vi "Fix up file date time to whats in file name.vi"(8 "error in":errorcluster) -> (0 "error out":errorcluster, 2 "Selected folder path":string, 3 "File path names":string[](array[string]))   [LabVIEW 2013]
panel:
  in  "Fix create date? (y)":bool=TRUE
  out "standard error":string
  out "standard output":string
  out "cmd shell cmds":string[](array[string])
  out "Records":i32
  # "Modified is false"
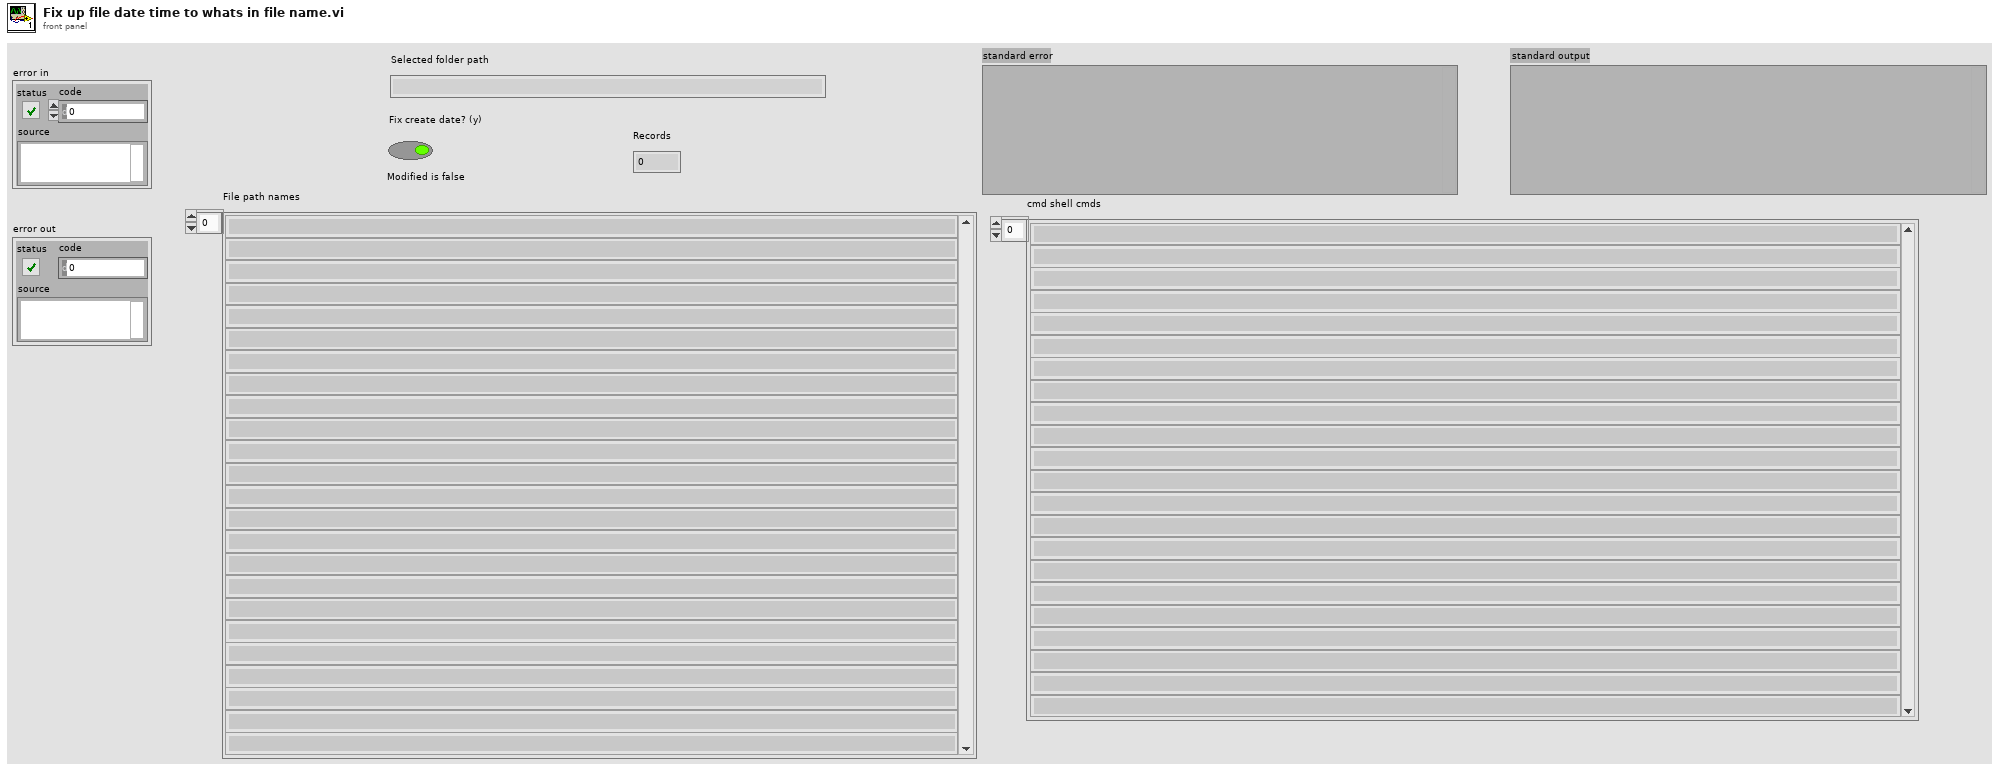
[diagram p1: front panel]
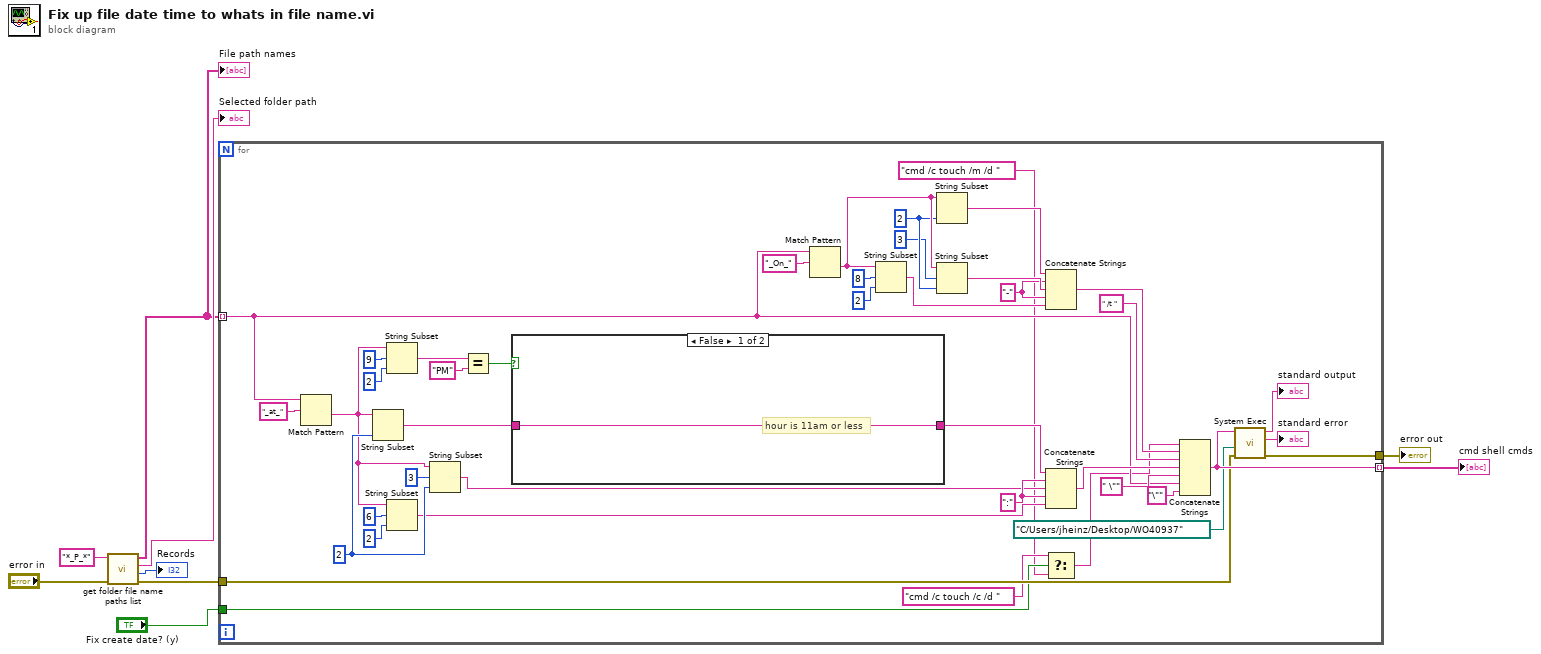
[diagram p0: block diagram]
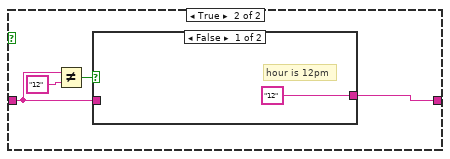
[diagram p2: hidden frame]
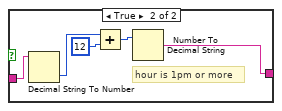
[diagram p3: hidden frame]
diagram:
  n1 = call "get folder file name paths list.vi"("error in"="error in", "file search pattern"="*_P_*") -> ("error out"=w4:errorcluster, "Records"=→"Records":i32, "Selected folder path"=→"Selected folder path":string, "File path names"=w5:string[])  [unwired: 6 in]
  "File path names" <- w5
  n2 = for {
    tunnel: w5 -> [w21] mode=indexing
    tunnel: w4 -> [w18]
    tunnel: [w17] -> w3
    tunnel: [w19] -> w2 mode=indexing
    tunnel: "Fix create date? (y)" -> [w13]
    w34 = ":" ("string")
    w37 = 2 ("length (rest)")
    w43 = "-" ("string")
    w49 = 2 ("length (rest)")
    n3 = Match Pattern(string=w21, regular expression="_at_") -> (after substring=w31:string)  [unwired: 1 in, 3 out]
    n4 = String Subset(string=w31, length (rest)=w37) -> (substring=w27:string)  [unwired: 1 in]
    n5 = String Subset(string=w31, offset (0)=9, length (rest)=2 ("length (rest)")) -> (substring=w30:string)
    n6 = String Subset(string=w31, offset (0)=6, length (rest)=2 ("length (rest)")) -> (substring=w32:string)
    n7 = String Subset(string=w31, offset (0)=3, length (rest)=w37) -> (substring=w33:string)
    n8 = Equal?(x=w30, y="PM") -> (x = y?=w28:bool)
    n9 = case shown="False" w28 {
      tunnel: w27 -> [w52 w54]
      tunnel: [w52 w53] -> w26
      frame False {
        # "hour is 11am or less"
      }
      frame True {
        n10 = Not Equal?(x=w54, y="12") -> (x != y?=w55:bool)
        n11 = case shown="False" w55 {
          tunnel: w54 -> [_ w62]
          tunnel: ["12" w58] -> w53
          frame False {
            # "hour is 12pm"
          }
          frame True {
            # "hour is 1pm or more"
            n12 = Decimal String To Number(string=w62) -> (number=w61:i32)  [unwired: 2 in, 1 out]
            n13 = Add(x=w61, y=12) -> (x+y=w59:i32)
            n14 = Number To Decimal String(number=w59) -> (decimal integer string=w58:string)  [unwired: 1 in]
          }
        }
      }
    }
    n15 = Match Pattern(string=w21, regular expression="_On_") -> (after substring=w50:string)  [unwired: 1 in, 3 out]
    n16 = String Subset(string=w50, offset (0)=8, length (rest)=2 ("length (rest)")) -> (substring=w42:string)
    n17 = String Subset(string=w50, length (rest)=w49) -> (substring=w45:string)  [unwired: 1 in]
    n18 = String Subset(string=w50, offset (0)=3, length (rest)=w49) -> (substring=w44:string)
    n19 = Concatenate Strings(w45, w43, w44, w43, w42) -> (w25:string)
    n20 = Concatenate Strings(w26, w34, w33, w34, w32) -> (w23:string)
    n21 = Select(t="cmd /c touch /c /d " ("string"), s=w13, f="cmd /c touch /m /d " ("string")) -> (s? t:f=w10:string)
    n22 = Concatenate Strings(w10, w25, " /t " ("string"), w23, " \"" ("string"), w21, "\"" ("string")) -> (w19:string)
    n23 = call <vilib>:"System Exec.vi"("error in (no error)"=w18, "working directory"=path "C:/Users/jheinz/Desktop/WO40937", "command line"=w19) -> ("error out"=w17:errorcluster, "standard error"=→"standard error":string, "standard output"=→"standard output":string)  [unwired: 5 in, 1 out]
  }
  "error out" <- w3
  "cmd shell cmds" <- w2
